vi "read_params.vi"(8 "error in (no error)":errorcluster, 11 "LassoLarsCV in":refnum<class "LassoLarsCV.lvclass">) -> (0 "error out":errorcluster, 2 "params":T1={"fit_intercept"=TRUE, "verbose"={"verbose_type"="bool", "verbose_bool"=FALSE, "verbose_int"=0.0}, "max_iter"=500.0, "normalize"=TRUE, "precompute"={"precompute_type"="auto", "precompute_bool"=FALSE, "precompute_list"=[]}, "cv"=5.0, "max_n_alphas"=1000.0, "n_jobs"=1.0, "copy_X"=TRUE, "positive"=FALSE}, 3 "LassoLarsCV out":refnum<class "LassoLarsCV.lvclass">)   [LabVIEW 2020, in "LassoLarsCV.lvclass"]
uses:
  LassoLarsCV.lvclass
  Controls/lasso_lars_cv_params.ctl
  LassoLarsCV.lvclass/LassoLarsCV.ctl
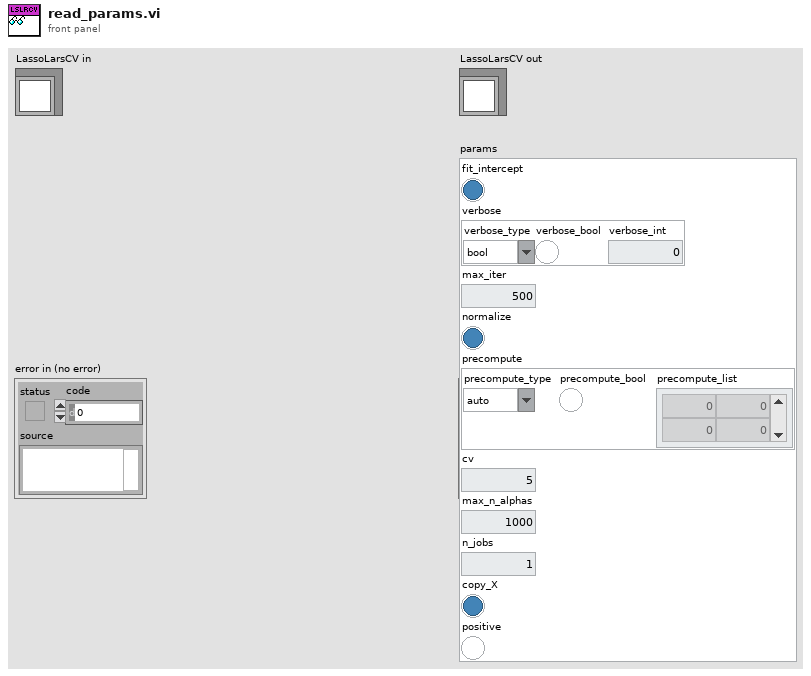
[diagram p1: front panel]
types:
  T1 = typedef "lasso_lars_cv_params.ctl" = cluster{"fit_intercept":bool, "verbose":cluster{"verbose_type":string, "verbose_bool":bool, "verbose_int":dbl}, "max_iter":dbl, "normalize":bool, "precompute":cluster{"precompute_type":string, "precompute_bool":bool, "precompute_list":dbl[][]}, "cv":dbl, "max_n_alphas":dbl, "n_jobs":dbl, "copy_X":bool, "positive":bool}
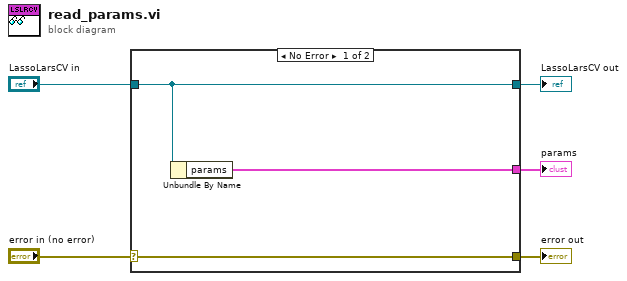
[diagram p0: block diagram]
diagram:
  n1 = case shown="No Error" "error in (no error)" {
    selector: "error in (no error)" -> [w8 w9]
    tunnel: [w8 w9] -> w4
    tunnel: [w7 w10] -> w2
    tunnel: "LassoLarsCV in" -> [w7 w10]
    tunnel: [w6 _] -> w1
    frame No Error {
      n2 = Unbundle By Name(w7) -> ("params"=w6:T1)
    }
    frame Error {
    }
  }
  "error out" <- w4
  "LassoLarsCV out" <- w2
  "params" <- w1
